vi "stepValueChanged.vi"(8 "error in (no error)":errorcluster, 9 "oldValue":dbl, 10 "newValue":dbl, 11 "ScanCreator in":refnum<class "ScanCreator.lvclass">) -> (0 "error out":errorcluster, 2 "passed":bool, 3 "ScanCreator out":refnum<class "ScanCreator.lvclass">)   [LabVIEW 2009, in "Views.lvlib" / "ScriptEditor.lvlib" / "ScanCreator.lvclass"]
uses:
  ScanCreator.lvclass
  ScanCreator.lvclass/ScanCreator.ctl
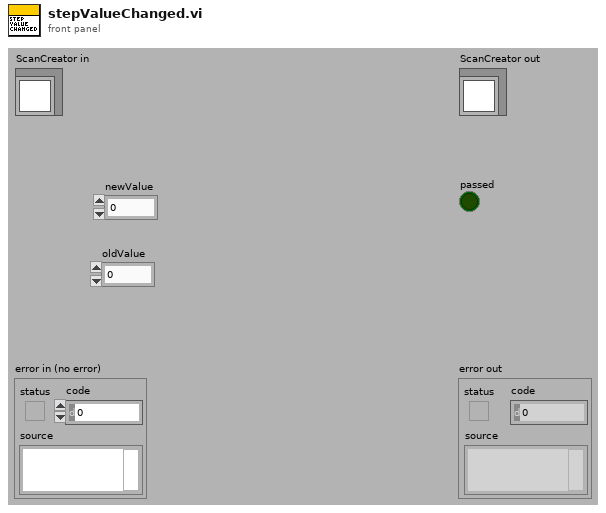
[diagram p1: front panel]
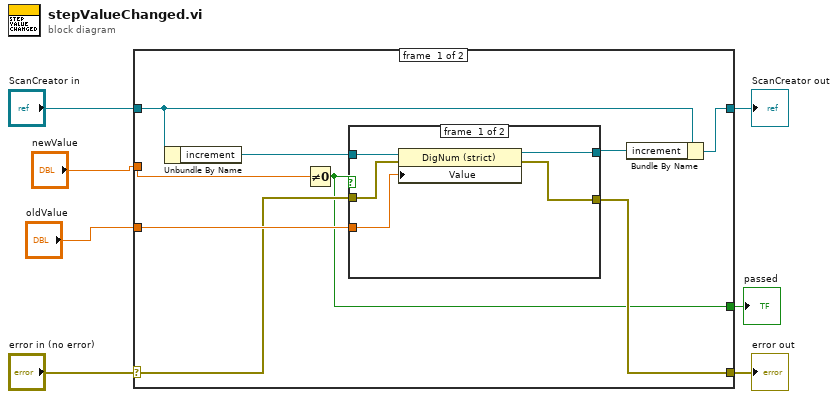
[diagram p0: block diagram]
diagram:
  n1 = case shown="No Error" "error in (no error)" {
    selector: "error in (no error)" -> [w11 w25]
    tunnel: [w10 w25] -> w6
    tunnel: [w8 w24] -> w4
    tunnel: "ScanCreator in" -> [w13 w24]
    tunnel: "newValue" -> [w16 _]
    tunnel: "oldValue" -> [w15 _]
    tunnel: [w9 _] -> w1
    frame #0 {
      n2 = Unbundle By Name(w13) -> ("increment"=w14:refnum<vi>)
      n3 = Not Equal To 0?(x=w16) -> (x != 0?=w9:bool)
      n4 = case shown="False" w9 {
        tunnel: w15 -> [w18 _]
        tunnel: w14 -> [w21 w23]
        tunnel: w11 -> [w20 w22]
        tunnel: [w19 w22] -> w10
        tunnel: [w17 w23] -> w12
        frame #0 {
          n5 = property class="DigNum (strict)"(reference=w21, error in=w20, "Value"=w18) -> (reference out=w17:refnum<vi>, error out=w19:errorcluster)
        }
        frame #1 {
        }
      }
      n6 = Bundle By Name(cluster=w13, "increment"=w12) -> (w8:refnum<class "ScanCreator.lvclass">)
    }
    frame #1 {
    }
  }
  "error out" <- w6
  "ScanCreator out" <- w4
  "passed" <- w1
